vi "PH_gentec_M-Link.Action get and set current Settings for the first Time.vi"(0 "i ref in":refnum<vi>, 5 "error in":errorcluster) -> (14 "i ref out":refnum<vi>, 19 "error out":errorcluster)   [LabVIEW 2014, in "PH_gentec_M-Link.lvlib"]
doc: "This VI gets and sets all current settings for the first time."
uses:
  PH_gentec_M-Link.lvlib
  non_GPL/instr.lib/gentec-M-LINK/Driver/Type Defs/gentec-M-Link.Measurement Mode.ctl
  non_GPL/instr.lib/gentec-M-LINK/Driver/Type Defs/gentec-M-Link.Range Queries.ctl
  non_GPL/instr.lib/gentec-M-LINK/Driver/Type Defs/gentec-M-Link.Trigger Source.ctl
  non_GPL/instr.lib/gentec-M-LINK/Driver/Type Defs/gentec-M-Link.Trigger Polarity.ctl
  PH_Powermeter_BaseClass/PH_Powermeter_BaseClass.State.ctl
  PH_Powermeter_BaseClass/PH_gentec_BaseClass.Head Settings.ctl
  non_GPL/instr.lib/gentec-M-LINK/gentec-M-Link - Driver.lvlib
  PH_Powermeter_BaseClass/PH_Powermeter_BaseClass.lvlib
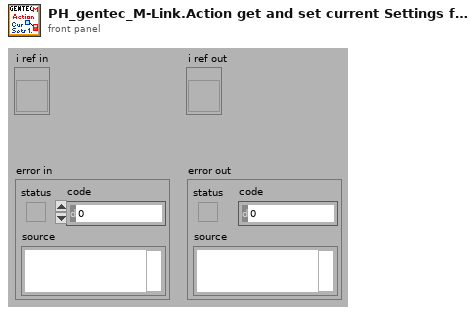
[diagram p1: front panel]
types:
  T1 = typedef "PH_Powermeter_BaseClass.lvlib/PH_gentec_BaseClass.Head Settings.ctl" = cluster{"Trigger Level":dbl, "Wavelength":u32, "Range":u32}
  T2 = typedef "PH_Powermeter_BaseClass.lvlib/PH_Powermeter_BaseClass.State.ctl" = enum32{"off", "operating", "opened", "checked", "connected", "Sets to change", "running"}
  T3 = typedef "gentec-M-Link - Driver.lvlib/gentec-M-Link.Range Queries.ctl" = string
  T4 = typedef "PH_Powermeter_BaseClass.lvlib/PH_Powermeter_BaseClass.i attribute.ctl" = cluster{"GUI References":T5, "Connection":T6, "Head Attributes":T7, "VISA resource":refnum<visa-resource-name>, "Energy":T8, "Service ID Energy":i32, "Wanted Settings":T1, "Current Settings":T1}
  T5 = typedef "PH_Powermeter_BaseClass.lvlib/PH_Powermeter_BaseClass.GUI Refs.ctl" = cluster{"Head Attributes":refnum<vi>, "Energy":refnum<vi>, "Connection":refnum<vi>, "VISA Resource":refnum<vi>, "Energy evolution":refnum<vi>, "Scaling Factor":refnum<vi>, "Range":refnum<vi>, "Wavelength":refnum<vi>, "Trigger Level":refnum<vi>, "Wanted Settings":refnum<vi>, "Current Settings":refnum<vi>}
  T6 = typedef "PH_Powermeter_BaseClass.lvlib/PH_Powermeter_BaseClass.Connection.ctl" = cluster{"failed checks":i8, "Timeout":bool, "Data read":string, "Failure":bool, "Error":bool, "State":T2}
  T7 = typedef "PH_Powermeter_BaseClass.lvlib/PH_Powermeter_BaseClass.Head Attributes.ctl" = cluster{"Instrument Type":string, "Head Version":string, "Head Name":string, "Serial Number":string, "Firmware":string, "Sensor Type":string, "MinimumRange":u32, "Maximum Range":u32, "Min Wavelength":i32, "Max Wavelength":i32}
  T8 = typedef "PH_Powermeter_BaseClass.lvlib/PH_Powermeter_BaseClass.Energy.ctl" = cluster{"current Value":dbl, "unscaled":dbl, "Scaling Factor":dbl}
  T9 = typedef "PH_gentec_M-Link.lvlib/PH_gentec_M-Link.i attribute.ctl" = cluster{"GUI References":cluster{"Wanted Head Settings":refnum<vi>, "Current Head Settings":refnum<vi>, "Set Auto Range":refnum<vi>, "Trigger Polarity":refnum<vi>, "Trigger Source":refnum<vi>, "Waveform Averages":refnum<vi>, "Continuous":refnum<vi>, "get one Value":refnum<vi>}, "Wanted Head Settings":T10, "Current Head Settings":T10}
  T10 = typedef "PH_gentec_M-Link.lvlib/PH_gentec_M-Link.Head Settings.ctl" = cluster{"Measurement Mode":T11, "Enable Anticipation":bool, "Set Auto Range":bool, "Block Signal":bool, "Set Head Attenuator":bool, "Enable SSE":bool, "Trigger Polarity":T12, "Trigger Source":T13, "Waveform Averages":T14, "Set Zero":i32, "Current Measurement":i32, "Start Data Flow":bool}
  T11 = typedef "gentec-M-Link - Driver.lvlib/gentec-M-Link.Measurement Mode.ctl" = u16
  T12 = typedef "gentec-M-Link - Driver.lvlib/gentec-M-Link.Trigger Polarity.ctl" = u16
  T13 = typedef "gentec-M-Link - Driver.lvlib/gentec-M-Link.Trigger Source.ctl" = u16
  T14 = typedef "gentec-M-Link - Driver.lvlib/gentec-M-Link.Waveform Averages.ctl" = u16
  T15 = typedef "gentec-M-Link - Driver.lvlib/gentec-M-Link.Range.ctl" = u16
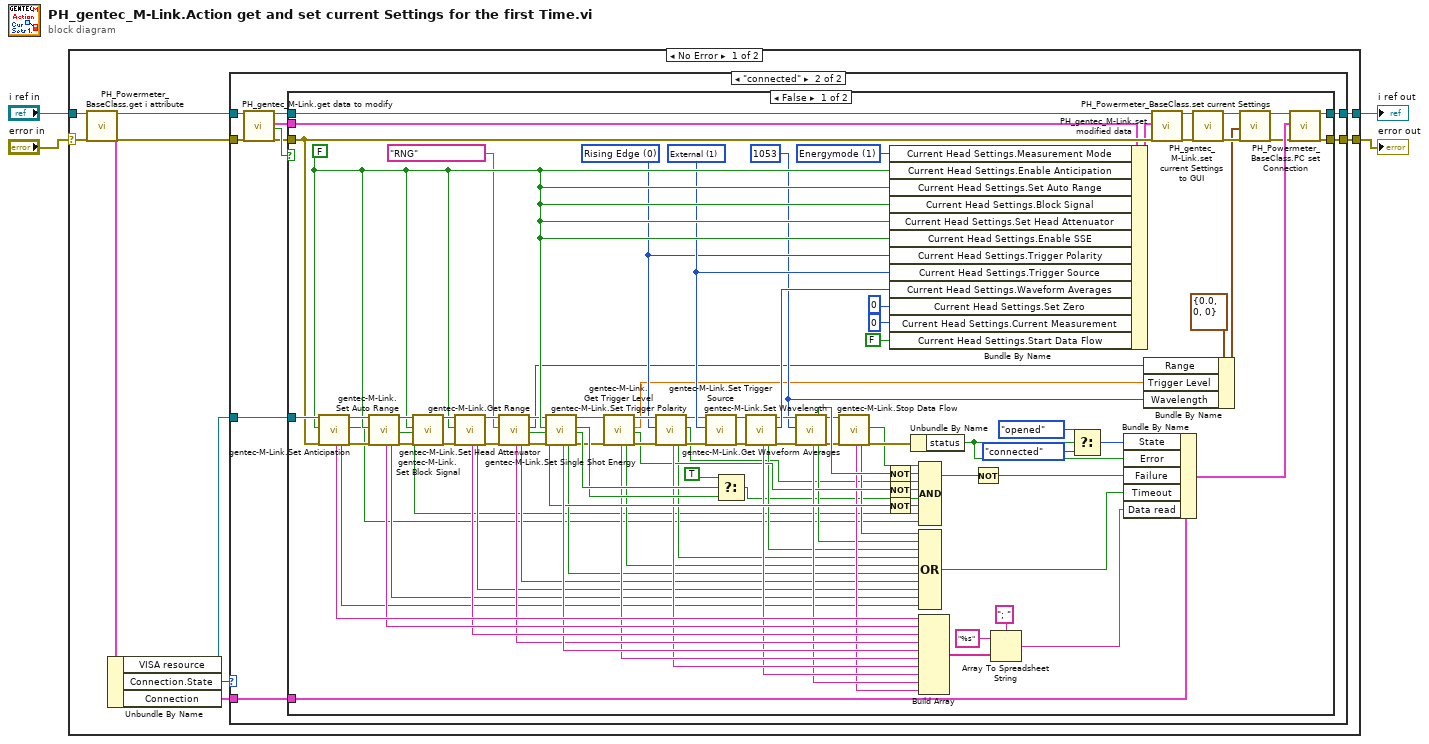
[diagram p0: block diagram]
diagram:
  n1 = case shown="No Error" "error in" {
    selector: "error in" -> [w5 w126]
    tunnel: [w14 w126] -> w4
    tunnel: [w13 w127] -> w3
    tunnel: "i ref in" -> [w12 w127]
    frame No Error {
      n2 = call "PH_Powermeter_BaseClass.get i attribute.vi"("i ref in"=w12, "error in (no error)"=w5) -> ("i ref out"=w8:refnum<vi>, "i attribute"=w11:T4, "error out"=w7:errorcluster)  [unwired: 15 in]
      n3 = Unbundle By Name(w11) -> ("VISA resource"=w6:refnum<visa-resource-name>, "Connection.State"=w10:T2, "Connection"=w9:T6)
      n4 = case shown="\"connected\"" w10 {
        tunnel: [w15 w17] -> w14
        tunnel: [w16 w18] -> w13
        tunnel: w6 -> [_ w22]
        tunnel: w8 -> [w16 w21]
        tunnel: w7 -> [w15 w20]
        tunnel: w9 -> [_ w19]
        frame Default {
        }
        frame "connected" {
          n5 = call "PH_gentec_M-Link.get data to modify.vi"("i ref in"=w21, "error in (no error)"=w20) -> ("i ref out"=w24:refnum<vi>, "i attribute"=w25:T9, "timed out"=w26:bool, "error out"=w23:errorcluster)  [unwired: 14 in]
          n6 = case shown="False" w26 {
            tunnel: w22 -> [w122 _]
            tunnel: [w40 w125] -> w18
            tunnel: [w39 w124] -> w17
            tunnel: w23 -> [w119 w124]
            tunnel: w24 -> [w123 w125]
            tunnel: w25 -> [w104 _]
            tunnel: w19 -> [w45 _]
            frame False {
              w29 = u16 1053 ("Lambda")
              w84 = T12 0 items=["Rising Edge", "Falling Edge"] ("Trigger Polarity")
              w89 = T13 1 items=["Internal", "External"] ("Trigger Source")
              w100 = FALSE ("Enable Anticipation")
              w103 = T11 1 items=["other Mode", "Energymode"] ("Measurement Mode")
              n7 = call "gentec-M-Link.Set Anticipation.vi"("VISA resource In"=w122, "Enable Anticipation"=w100, "error in (no error)"=w119) -> ("Data Read"=w114:string, "Read Timeout"=w58:bool, "VISA resource Out"=w120:refnum<visa-resource-name>, "Success"=w50:bool, "error out"=w118:errorcluster)  [unwired: 12 in]
              n8 = call "gentec-M-Link.Set Auto Range.vi"("VISA resource In"=w120, "Auto Range"=w100, "error in (no error)"=w118) -> ("Data Read"=w113:string, "Read Timeout"=w59:bool, "VISA resource Out"=w121:refnum<visa-resource-name>, "Success"=w51:bool, "error out"=w117:errorcluster)  [unwired: 12 in]
              n9 = call "gentec-M-Link.Set Block Signal.vi"("VISA resource In"=w121, "Block Signal"=w100, "error in (no error)"=w117) -> ("VISA resource Out"=w116:refnum<visa-resource-name>, "error out"=w115:errorcluster)  [unwired: 15 in]
              n10 = call "gentec-M-Link.Set Head Attenuator.vi"("VISA resource In"=w116, "Set Head Attenuator"=w100, "error in (no error)"=w115) -> ("Data Read"=w112:string, "Read Timeout"=w60:bool, "VISA resource Out"=w99:refnum<visa-resource-name>, "error out"=w97:errorcluster)  [unwired: 11 in, 2 out]
              n11 = call "gentec-M-Link.Get Range.vi"("VISA resource In"=w99, "Range Queries"=T3 "RNG", "error in (no error)"=w97) -> ("Data Read"=w94:string, "Read Timeout"=w61:bool, "VISA resource Out"=w98:refnum<visa-resource-name>, "Range"=w27:T15, "Error"=w93:bool, "error out"=w96:errorcluster)  [unwired: 11 in]
              n12 = call "gentec-M-Link.Set Single Shot Energy.vi"("VISA resource In"=w98, "Enable Single Shot Energy"=w100, "error in (no error)"=w96) -> ("Data Read"=w111:string, "Read Timeout"=w62:bool, "VISA resource Out"=w92:refnum<visa-resource-name>, "Success"=w106:bool, "no Thermopyle Head"=w107:bool, "error out"=w91:errorcluster)  [unwired: 11 in]
              n13 = call "gentec-M-Link.Get Trigger Level.vi"("VISA resource In"=w92, "error in (no error)"=w91) -> ("Data Read"=w90:string, "Read Timeout"=w63:bool, "VISA resource Out"=w86:refnum<visa-resource-name>, "Trigger Level [%]"=w28:dbl, "Error"=w74:bool, "error out"=w88:errorcluster)  [unwired: 12 in]
              n14 = call "gentec-M-Link.Set Trigger Polarity.vi"("VISA resource In"=w86, "Trigger Polarity"=w84, "error in (no error)"=w88) -> ("Data Read"=w83:string, "Read Timeout"=w64:bool, "VISA resource Out"=w85:refnum<visa-resource-name>, "Success"=w55:bool, "error out"=w87:errorcluster)  [unwired: 12 in]
              n15 = call "gentec-M-Link.Set Trigger Source.vi"("VISA resource In"=w85, "Trigger Source"=w89, "error in (no error)"=w87) -> ("VISA resource Out"=w82:refnum<visa-resource-name>, "error out"=w81:errorcluster)  [unwired: 15 in]
              n16 = Select(t=TRUE, s=w107, f=w106) -> (s? t:f=w53:bool)
              n17 = call "gentec-M-Link.Get Waveform Averages.vi"("VISA resource In"=w82, "error in (no error)"=w81) -> ("Data Read"=w80:string, "Read Timeout"=w65:bool, "VISA resource Out"=w77:refnum<visa-resource-name>, "Waveform Averages"=w79:T14, "error out"=w78:errorcluster)  [unwired: 13 in]
              n18 = call "gentec-M-Link.Set Wavelength.vi"("VISA resource In"=w77, "Lambda"=w29, "error in (no error)"=w78) -> ("Data Read"=w76:string, "Error"=w75:bool, "Read Timeout"=w66:bool, "VISA resource Out"=w71:refnum<visa-resource-name>, "error out"=w73:errorcluster)  [unwired: 8 in, 4 out]
              n19 = call "gentec-M-Link.Stop Data Flow.vi"("VISA resource In"=w71, "error in (no error)"=w73) -> ("Data Read"=w68:string, "Read Timeout"=w67:bool, "Success"=w57:bool, "error out"=w72:errorcluster)  [unwired: 13 in, 1 out]
              n20 = Not(x=w75) -> (.not. x?=w56:bool)
              n21 = Not(x=w74) -> (.not. x?=w54:bool)
              n22 = Not(x=w93) -> (.not. x?=w52:bool)
              n23 = Bundle By Name(cluster=w104, "Current Head Settings.Measurement Mode"=w103, "Current Head Settings.Enable Anticipation"=w100, "Current Head Settings.Set Auto Range"=w100, "Current Head Settings.Block Signal"=w100, "Current Head Settings.Set Head Attenuator"=w100, "Current Head Settings.Enable SSE"=w100, "Current Head Settings.Trigger Polarity"=w84, "Current Head Settings.Trigger Source"=w89, "Current Head Settings.Waveform Averages"=w79, "Current Head Settings.Set Zero"=0, "Current Head Settings.Current Measurement"=0, "Current Head Settings.Start Data Flow"=FALSE) -> (w102:T9)
              n24 = Unbundle By Name(w72) -> ("status"=w43:bool)
              n25 = Compound Arithmetic op=AND(w57, w56, w55, w54, w53, w52, w51, w50) -> (w49:bool)
              n26 = Compound Arithmetic op=OR(w67, w66, w65, w64, w63, w62, w61, w60, w59, w58) -> (w47:bool)
              n27 = Build Array(w114, w113, w112, w94, w111, w90, w83, w80, w76, w68) -> (w108:string[])
              n28 = Not(x=w49) -> (.not. x?=w46:bool)
              n29 = Array To Spreadsheet String(delimiter (Tab)="; ", array=w108, 3:"%s" ("format string")) -> (spreadsheet string=w48:string)
              n30 = Select(t=PH_Powermeter_BaseClass.State."opened" ("State"), s=w43, f=PH_Powermeter_BaseClass.State."connected") -> (s? t:f=w41:T2)
              n31 = Bundle By Name(cluster=w45, "State"=w41, "Error"=w43, "Failure"=w46, "Timeout"=w47, "Data read"=w48) -> (w38:T6)
              n32 = Bundle By Name(cluster=T1 {"Trigger Level"=0.0, "Wavelength"=0, "Range"=0} ("Current Settings"), "Range"=w27, "Trigger Level"=w28, "Wavelength"=w29) -> (w30:T1)
              n33 = call "PH_gentec_M-Link.set modified data.vi"("i ref in"=w123, "i attribute"=w102, "error in (no error)"=w119) -> ("i ref out"=w37:refnum<vi>, "error out"=w36:errorcluster)  [unwired: 15 in]
              n34 = call "PH_gentec_M-Link.set current Settings to GUI.vi"("i ref in"=w37, "error in"=w36) -> ("i ref out"=w33:refnum<vi>, "error out"=w35:errorcluster)  [unwired: 16 in]
              n35 = call "PH_Powermeter_BaseClass.set current Settings.vi"("VI in"=w33, "Current Settings"=w30, "error in (no error)"=w35) -> ("VI out"=w32:refnum<vi>, "error out"=w34:errorcluster)  [unwired: 15 in]
              n36 = call "PH_Powermeter_BaseClass.PC set Connection.vi"("VI in"=w32, "Connection"=w38, "error in (no error)"=w34) -> ("VI out"=w40:refnum<vi>, "error out"=w39:errorcluster)  [unwired: 15 in]
            }
            frame True {
            }
          }
        }
      }
    }
    frame Error {
    }
  }
  "error out" <- w4
  "i ref out" <- w3
